vi "Average 2D Array to 1D Array.vi"(11 "Array":dbl[][](array[numeric])) -> (3 "Array 2":dbl[](array[numeric]))   [LabVIEW 2018]
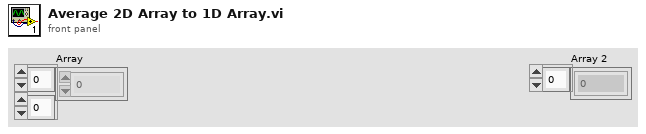
[diagram p1: front panel]
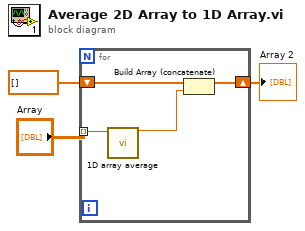
[diagram p0: block diagram]
diagram:
  n1 = for {
    shift-right: [w6] -> w1
    shift-left: dbl[] [] -> [w7]
    tunnel: "Array" -> [w5] mode=indexing
    n2 = call "1D array average.vi"("Array"=w5) -> ("Output"=w4:dbl)  [unwired: 10 in]
    n3 = Build Array (concatenate)(w7, w4) -> (w6:dbl[])
  }
  "Array 2" <- w1
